vi "set_data_exp.vi"(8 "error in (no error)":errorcluster, 10 "Data":dbl[][](array[numeric]), 11 "Experiment.lvclass in":refnum<class "Experiment.lvclass">) -> (0 "error out":errorcluster, 3 "Experiment.lvclass out":refnum<class "Experiment.lvclass">)   [LabVIEW 2015, in "Experiment.lvclass"]
uses:
  Experiment.lvclass
  Experiment.lvclass/Experiment.ctl
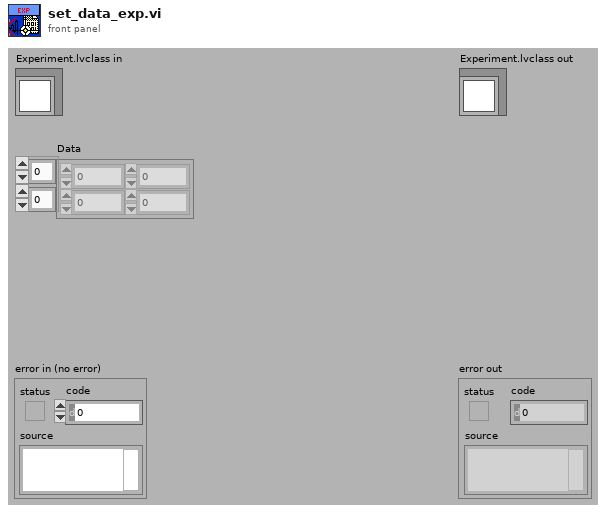
[diagram p1: front panel]
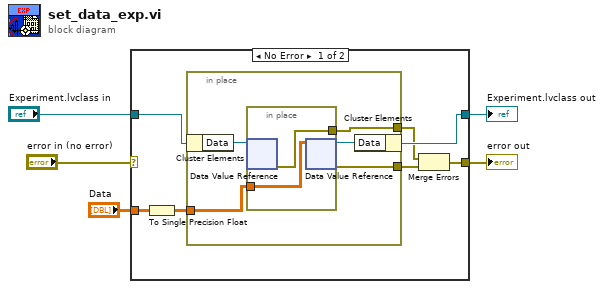
[diagram p0: block diagram]
diagram:
  n1 = case shown="No Error" "error in (no error)" {
    selector: "error in (no error)" -> [_ w20]
    tunnel: [w8 w20] -> w4
    tunnel: [w10 w21] -> w2
    tunnel: "Experiment.lvclass in" -> [w11 w21]
    tunnel: "Data" -> [w12 _]
    frame No Error {
      n2 = To Single Precision Float(number=w12) -> (single precision float=w9:sgl[][])
      n3 = in-place {
        in-place-border: w9 -> [w16]
        in-place-border: [w14] -> w7
        in-place-border: [w13] -> w6
        n4 = in-place-cluster #1(w11) -> ("Data"=w17:refnum<data-value>)
        n5 = in-place {
          in-place-border: w16 -> [w19]
          in-place-border: [w18] -> w13
          n6 = in-place-dvr #2(w17) -> (w18:errorcluster)  [unwired: 1 out]
          n7 = in-place-dvr #2(w19) -> (w15:refnum<data-value>, w14:errorcluster)
        }
        n8 = in-place-cluster #1("Data"=w15) -> (w10:refnum<class "Experiment.lvclass">)
      }
      n9 = Merge Errors(w6, w7) -> (w8:errorcluster)
    }
    frame Error {
    }
  }
  "error out" <- w4
  "Experiment.lvclass out" <- w2
